vi "Global Zero Constants.vi"() -> ()   [LabVIEW 2020]
panel:
  in  "Zero Constants":dbl[](array[numeric])
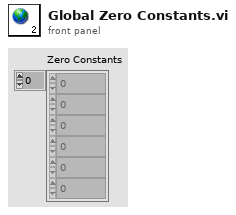
[diagram p1: front panel]
diagram:
